vi "lettura V-I ac&dc.vi"(8 "error in (no error)":errorcluster, 11 "Refnum in":refnum<k21>) -> (0 "error out":errorcluster, 1 "Cluster":T1, 2 "fc - Sampling frequency \nof the card":dbl=50000.0, 3 "Refnum out":refnum<k21>)   [LabVIEW 2018]
uses:
  <vilib>/DAQmx/read.llb/DAQmx Read (Analog 2D DBL NChan NSamp).vi
  coppie.ctl
  array misure.ctl
  <resource>/objmgr/daqmx.rc
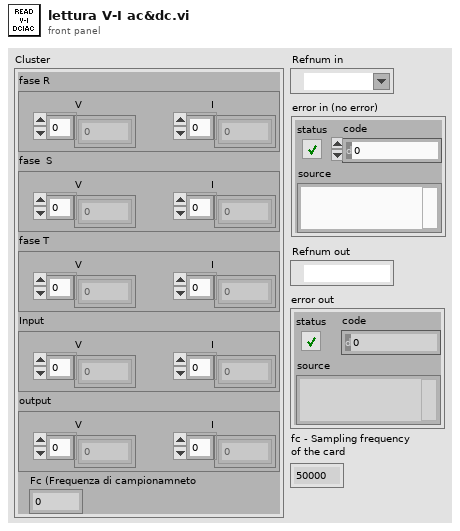
[diagram p1: front panel]
types:
  T1 = typedef "array misure.ctl" = cluster{"fase R ":T2, "fase  S":T2, "fase T":T2, "Input":T2, "output":T2, "Fc (Frequenza di campionamneto":dbl}
  T2 = typedef "coppie.ctl" = cluster{"V":dbl[], "I":dbl[]}
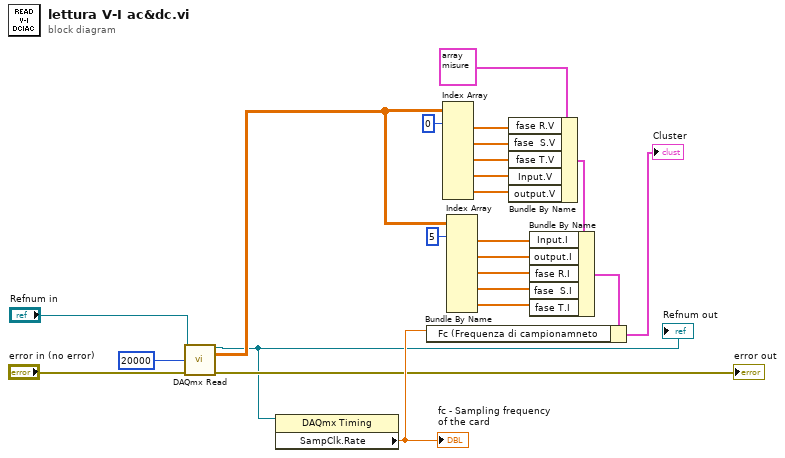
[diagram p0: block diagram]
diagram:
  n1 = call-poly <vilib>:"DAQmx Read.vi"("task/channels in"="Refnum in", "number of samples per channel"=20000, "error in"="error in (no error)") -> ("task out"=w1:refnum<k21>, "data"=w10:dbl[][], "error out"=→"error out":errorcluster)  [unwired: 10 in]
  "Refnum out" <- w1
  n2 = property class="DAQmx Timing"(reference=w1) -> ("SampClk.Rate"=w20:dbl)  [unwired: 1 in, 2 out]
  "fc - Sampling frequency \nof the card" <- w20
  n3 = Index Array(array=w10, index (row) #1=0 ("index (row)")) -> (element #1=w4:dbl[], element #2=w5:dbl[], element #3=w6:dbl[], element #4=w7:dbl[], element #5=w8:dbl[])  [unwired: 9 in]
  n4 = Index Array(array=w10, index (row) #1=5 ("index (row)")) -> (element #1=w12:dbl[], element #2=w13:dbl[], element #3=w14:dbl[], element #4=w23:dbl[], element #5=w21:dbl[])  [unwired: 9 in]
  n5 = Bundle By Name(cluster=T1 {"fase R "={"V"=[], "I"=[]}, "fase  S"={"V"=[], "I"=[]}, "fase T"={"V"=[], "I"=[]}, "Input"={"V"=[], "I"=[]}, "output"={"V"=[], "I"=[]}, "Fc (Frequenza di campionamneto"=0.0} ("Cluster"), "fase R.V"=w4, "fase  S.V"=w5, "fase T.V"=w6, "Input.V"=w7, "output.V"=w8) -> (w15:T1)
  n6 = Bundle By Name(cluster=w15, "Input.I"=w12, "output.I"=w13, "fase R.I"=w14, "fase  S.I"=w23, "fase T.I"=w21) -> (w19:T1)
  n7 = Bundle By Name(cluster=w19, "Fc (Frequenza di campionamneto"=w20) -> (→"Cluster":T1)
